vi "Populate Missing Bus Voltages.vi"(7 "Network Data Array":T1[](array[typedef]), 8 "error in":errorcluster, 11 "Bus Voltage Array in":T2[](array[typedef])) -> (0 "error out":errorcluster, 3 "Bus Voltage Array out":T2[](array[typedef]))   [LabVIEW 2018, in "Generic Optimization Actor.lvlib" / "Generic Optimization.lvclass"]
uses:
  Generic Optimization.lvclass
  Optimization Controls/Bus Voltage.ctl
  Optimization Controls/Electrical Network Optimization Data.ctl
  <vilib>/Analysis/NI_AALBase.lvlib
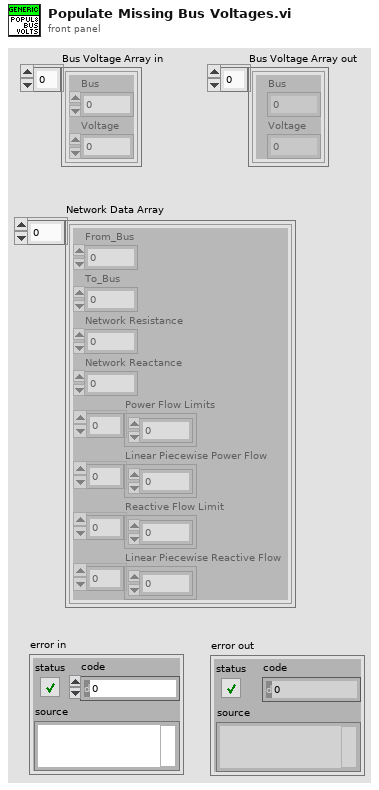
[diagram p1: front panel]
types:
  T1 = typedef "Generic Optimization Actor.lvlib/Generic Optimization.lvclass/Electrical Network Optimization Data.ctl" = cluster{"From_Bus":dbl, "To_Bus":dbl, "Network Resistance":dbl, "Network Reactance":dbl, "Power Flow Limits":dbl[], "Linear Piecewise Power Flow":dbl[], "Reactive Flow Limit":dbl[], "Linear Piecewise Reactive Flow":dbl[]}
  T2 = typedef "Generic Optimization Actor.lvlib/Generic Optimization.lvclass/Bus Voltage.ctl" = cluster{"Bus":dbl, "Voltage":dbl}
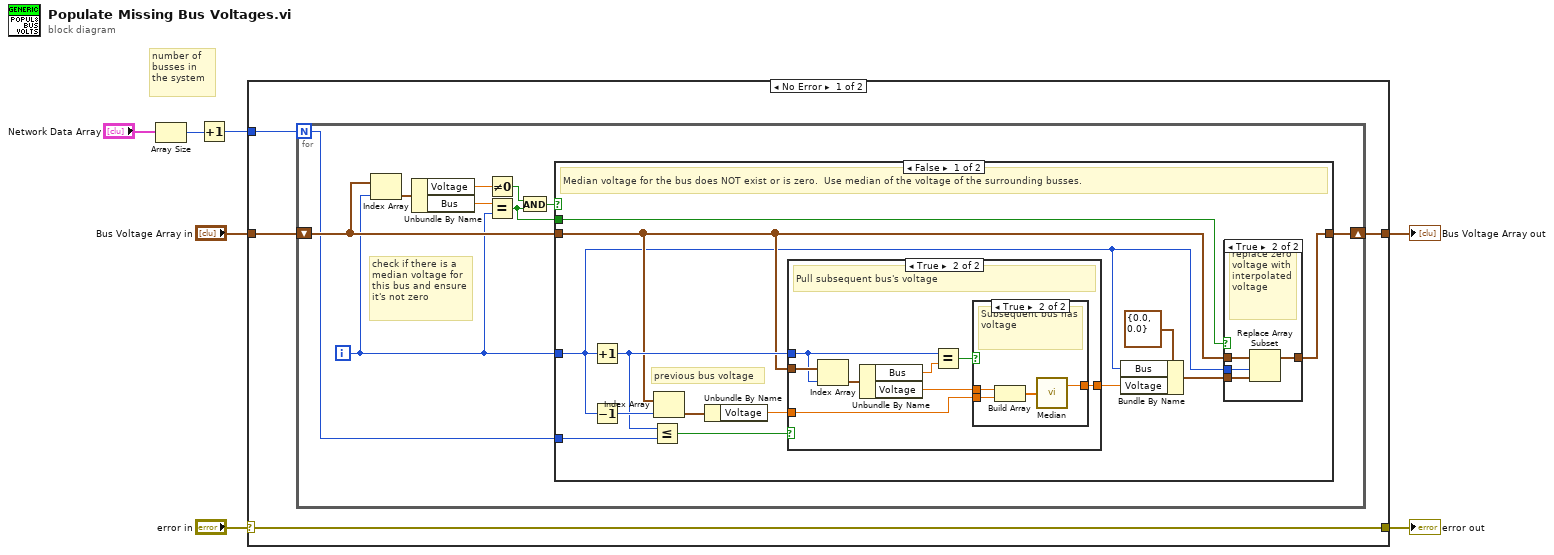
[diagram p0: block diagram]
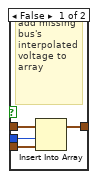
[diagram p2: hidden frame]
diagram:
  # "number of busses in the system"
  n1 = Array Size(array="Network Data Array") -> (size(s)=w2:i32)
  n2 = Increment(x=w2) -> (x+1=w1:i32)
  n3 = case shown="No Error" "error in" {
    selector: "error in" -> [w8 w58]
    tunnel: [w11 w59] -> w7
    tunnel: w1 -> [w10 _]
    tunnel: "Bus Voltage Array in" -> [w9 w59]
    tunnel: [w8 w58] -> w4
    frame No Error {
      n4 = for {
        N: w10 -> [w16]
        shift-right: [w18] -> w11
        shift-left: w9 -> [w20]
        i -> [w17]
        # "check if there is a median voltage for this bus and ensure it's not zero"
        n5 = Index Array(array=w20, index=w17) -> (element=w19:T2)
        n6 = Unbundle By Name(w19) -> ("Voltage"=w15:dbl, "Bus"=w21:dbl)
        n7 = Not Equal To 0?(x=w15) -> (x != 0?=w14:bool)
        n8 = Equal?(x=w21, y=w17) -> (x = y?=w12:bool)
        n9 = And(x=w14, y=w12) -> (x .and. y?=w13:bool)
        n10 = case shown="False" w13 {
          tunnel: w20 -> [w29 w57]
          tunnel: [w24 w57] -> w18
          tunnel: w17 -> [w25 _]
          tunnel: w16 -> [w31 _]
          tunnel: w12 -> [w22 _]
          frame False {
            # "previous bus voltage"
            # "Median voltage for the bus does NOT exist or is zero.  Use median of the voltage of the surrounding busses."
            n11 = Increment(x=w25) -> (x+1=w32:i32)
            n12 = Decrement(x=w25) -> (x-1=w34:i32)
            n13 = Less Or Equal?(x=w32, y=w31) -> (x <= y?=w30:bool)
            n14 = Index Array(array=w29, index=w34) -> (element=w28:T2)
            n15 = Unbundle By Name(w28) -> ("Voltage"=w33:dbl)
            n16 = case shown="True" w30 {
              tunnel: w29 -> [_ w50]
              tunnel: w33 -> [w43 w48]
              tunnel: w32 -> [_ w45]
              tunnel: [w43 w47] -> w27
              frame False {
                # "This is the last bus.  Use previous bus voltage."
              }
              frame True {
                # "Pull subsequent bus's voltage"
                n17 = Index Array(array=w50, index=w45) -> (element=w51:T2)
                n18 = Unbundle By Name(w51) -> ("Bus"=w46:dbl, "Voltage"=w49:dbl)
                n19 = Equal?(x=w45, y=w46) -> (x = y?=w44:bool)
                n20 = case shown="True" w44 {
                  tunnel: w49 -> [_ w56]
                  tunnel: w48 -> [w52 w55]
                  tunnel: [w52 w53] -> w47
                  frame False {
                    # "No voltage on subsequent bus"
                  }
                  frame True {
                    # "Subsequent bus has voltage"
                    n21 = Build Array(w56, w55) -> (w54:dbl[])
                    n22 = call <vilib>:"Median.vi"("X"=w54) -> ("median"=w53:dbl)  [unwired: 1 out]
                  }
                }
              }
            }
            n23 = Bundle By Name(cluster=T2 {"Bus"=0.0, "Voltage"=0.0} ("Bus Voltage"), "Bus"=w25, "Voltage"=w27) -> (w26:T2)
            n24 = case shown="True" w22 {
              tunnel: w29 -> [w38 w42]
              tunnel: w26 -> [w37 w41]
              tunnel: w25 -> [w36 w40]
              tunnel: [w35 w39] -> w24
              frame False {
                # "add missing bus's interpolated voltage to array"
                n25 = Insert Into Array(array=w38, index=w36, new element=w37) -> (w35:T2[])
              }
              frame True {
                # "replace zero voltage with interpolated voltage"
                n26 = Replace Array Subset(array=w42, new element=w41, index=w40) -> (w39:T2[])
              }
            }
          }
          frame True {
            # "Mean voltage for this bus already exists.  Do nothing."
          }
        }
      }
    }
    frame Error {
    }
  }
  "Bus Voltage Array out" <- w7
  "error out" <- w4
